vi "Get Reference.vi"(8 "error in (no error)":errorcluster, 10 "Name":string, 11 "UI Reference Wrapper in":refnum<class "UI Reference Wrapper.lvclass">) -> (0 "error out":errorcluster, 1 "VI Refnum":refnum<vi>, 2 "key not found?":bool, 3 "UI Reference Wrapper out":refnum<class "UI Reference Wrapper.lvclass">)   [LabVIEW 2020, in "UI Reference Wrapper.lvclass"]
uses:
  UI Reference Wrapper.lvclass
  UI Reference Wrapper.lvclass/UI Reference Wrapper.ctl
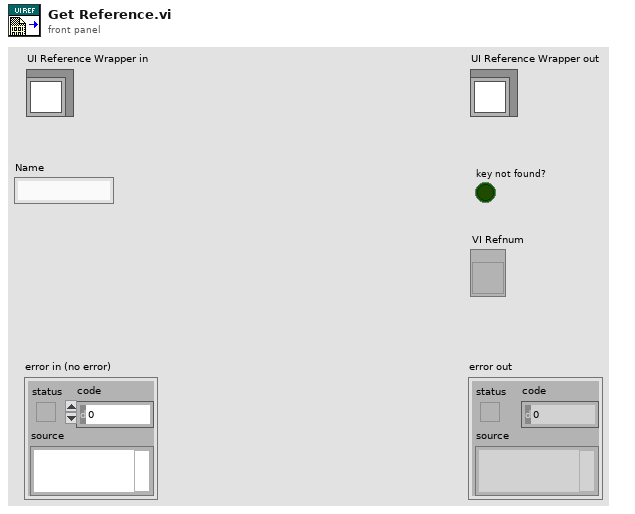
[diagram p1: front panel]
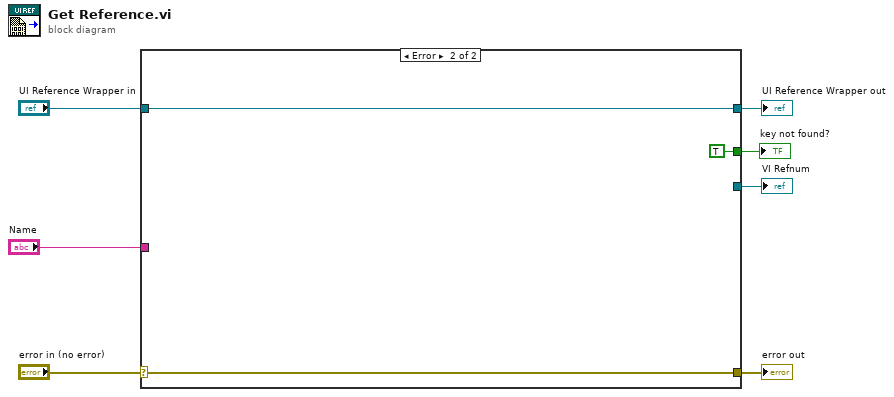
[diagram p0: block diagram]
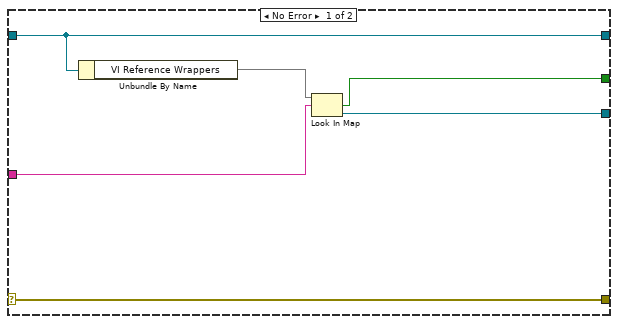
[diagram p2: hidden frame]
diagram:
  n1 = case shown="Error" "error in (no error)" {
    selector: "error in (no error)" -> [w13 w16]
    tunnel: [w13 w16] -> w6
    tunnel: [w12 w15] -> w4
    tunnel: "UI Reference Wrapper in" -> [w12 w15]
    tunnel: "Name" -> [w10 _]
    tunnel: [w9 _] -> w2
    tunnel: [w8 TRUE ("key not found?")] -> w1
    frame No Error {
      n2 = Unbundle By Name(w12) -> ("VI Reference Wrappers"=w11:map{string, refnum<vi>})
      n3 = Look In Map(map=w11, key=w10) -> (key not found?=w8:bool, value=w9:refnum<vi>)  [unwired: 1 in]
    }
    frame Error {
    }
  }
  "error out" <- w6
  "UI Reference Wrapper out" <- w4
  "VI Refnum" <- w2
  "key not found?" <- w1
